vi "ex9-2.vi"() -> ()   [LabVIEW 2013]
panel:
  out "Steering":i32=100
  in  "Steering":dbl(slide) scale=-100.0..100.0
  in  "Power":dbl(slide) scale=-100.0..100.0
  out "Power":i32=75
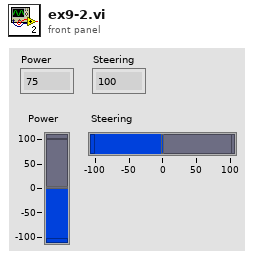
[diagram p1: front panel]
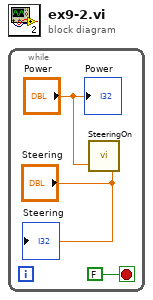
[diagram p0: block diagram]
diagram:
  n1 = while {
    stop <- FALSE stop-if-true
    n2 = call <vilib>:"SteeringOn.vi"("Power (75)"="Power", "Steering (100)"="Steering") -> ()  [unwired: 2 in, 1 out]
    "Power" <- "Power"
    "Steering" <- "Steering"
  }
